vi "ClearDTCs.vi"(8 "error in (no error)":errorcluster, 9 "timeout ms (1000)":i32=1000, 10 "Options (KWP/UDS Only)":T1={"Group of DTC"=16777215, "Byte Lengths"={"Override"=FALSE, "DTC"=0, "Status"=0, "Failure"=0}} {"Group of DTC" format="%.0x"}, 11 "Ref":T3) -> (0 "error out":errorcluster, 3 "Ref":T3)   [LabVIEW 2019, in "Diagnostics Host Automation API.lvlib"]
uses:
  Diagnostics Host Automation API.lvlib
  Addon/Addon Shared/Types/HostAutomation.Ref.ctl
  <vilib>/NI/STM/TCP/TCP Connection Info.ctl
  <vilib>/NI/STM/SubVIs/MetaDataElement.ctl
  Addon/Addon Shared/Types/DTC.Codes.ctl
  Addon/Addon Shared/Types/Command.ClearDTC.ctl
  Addon/Addon Shared/Types/DTC.Descriptor.Override.ctl
  <vilib>/NI/NI VeriStand Addon Network Comm/Shared/NI VeriStand Addon Network Comm Shared.lvlib
  <vilib>/NI/STM/NI STM.lvlib
  Addon/Addon Shared/Diagnostics Addon Shared.lvlib
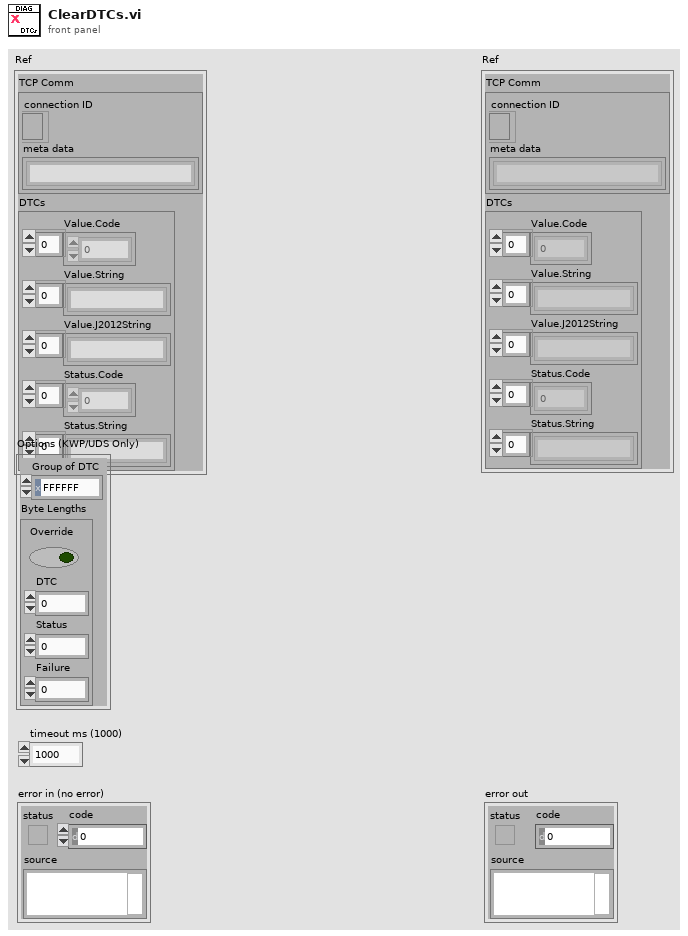
[diagram p1: front panel]
types:
  T1 = typedef "Diagnostics Addon Shared.lvlib/Command.ClearDTC.ctl" = cluster{"Group of DTC":u32, "Byte Lengths":T2}
  T2 = typedef "Diagnostics Addon Shared.lvlib/DTC.Descriptor.Override.ctl" = cluster{"Override":bool, "DTC":u32, "Status":u32, "Failure":u32}
  T3 = typedef "Diagnostics Addon Shared.lvlib/HostAutomation.Ref.ctl" = cluster{"TCP Comm":T4, "DTCs":T6}
  T4 = typedef "NI STM.lvlib/TCP Connection Info.ctl" = cluster{"connection ID":refnum<k5>, "meta data":T5[]}
  T5 = typedef "NI STM.lvlib/MetaDataElement.ctl" = string
  T6 = typedef "Diagnostics Addon Shared.lvlib/DTC.Codes.ctl" = cluster{"Value.Code":dbl[], "Value.String":string[], "Value.J2012String":string[], "Status.Code":dbl[], "Status.String":string[]}
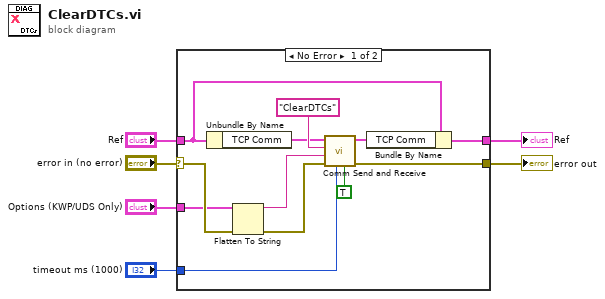
[diagram p0: block diagram]
diagram:
  n1 = case shown="No Error" "error in (no error)" {
    selector: "error in (no error)" -> [w18 w20]
    tunnel: "Ref" -> [w9 w19]
    tunnel: [w7 w19] -> w5
    tunnel: [w12 w20] -> w4
    tunnel: "timeout ms (1000)" -> [w14 _]
    tunnel: "Options (KWP/UDS Only)" -> [w17 _]
    frame No Error {
      n2 = Unbundle By Name(w9) -> ("TCP Comm"=w10:T4)
      n3 = Flatten To String(anything=w17, error in (no error)=w18) -> (data string=w15:string, error out=w11:errorcluster)  [unwired: 2 in, 1 out]
      n4 = call <vilib>:"Comm Send and Receive.vi"("Resp Required?"=TRUE, "Timeout (ms)"=w14, "error in (no error)"=w11, "Data"=w15, "Name"="ClearDTCs", "connection info"=w10) -> ("error out"=w12:errorcluster, "connection info"=w8:T4)  [unwired: 2 in, 2 out]
      n5 = Bundle By Name(cluster=w9, "TCP Comm"=w8) -> (w7:T3)
    }
    frame Error {
    }
  }
  "Ref" <- w5
  "error out" <- w4
